vi "VI Tree.vi"   [LabVIEW 2016, in "Tektronix DPO MSO 2000 4000 Series.lvlib"]
doc: "This is the instrument driver for Tektronix DPO (2k, 3k, 4k), MSO (2k, 3k, 4k), and MDO. The VI Tree displays all the user-callable VIs of the instrument driver in an organized table."
uses:
  Tektronix DPO MSO 2000 4000 Series.lvlib
  Configure/Configure Probe (Auxiliary).vi
  Data/Data_Low Level/Fetch Waveform (Waveform Data Type).vi
  Configure/Configure Math (Dual).vi
  Configure/Configure Trigger (USB).vi
  Configure/Configure Bus Source (I2C).vi
  Data/Read (Multiple Waveforms).vi
panel:
  # "(C) 2006 - 2016. National Instruments Corporation. ALL RIGHTS RESERVED."
  # "SEE DIAGRAM\nFOR VI TREE."
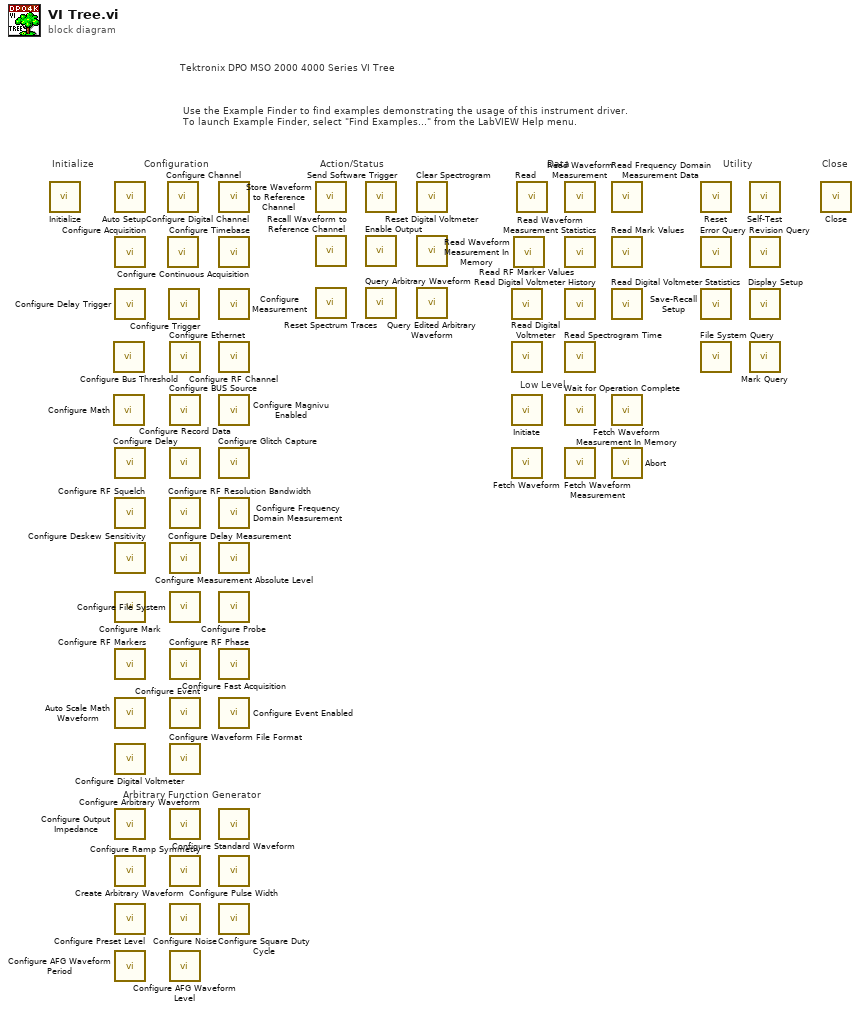
[diagram p0: block diagram]
diagram:
  # "Arbitrary Function Generator"
  # "Tektronix DPO MSO 2000 4000 Series VI Tree"
  # "Use the Example Finder to find examples demonstrating the usage of this instrument driver.\nTo launch Example Finder, select \"Find Examples...\" from the LabVIEW Help menu."
  # "Low Level"
  # "Action/Status"
  # "Configuration"
  # "Utility"
  # "Data"
  # "Close"
  # "Initialize"
  n1 = call "Initialize.vi"() -> ()  [unwired: 10 in, 2 out]
  n2 = call "Configure Bus Threshold.vi"() -> ()  [unwired: 10 in, 2 out]
  n3 = call-poly "Configure Math.vi"() -> ()  [unwired: 10 in, 2 out]
  n4 = call "Auto Setup.vi"() -> ()  [unwired: 10 in, 2 out]
  n5 = call "Configure Acquisition.vi"() -> ()  [unwired: 10 in, 2 out]
  n6 = call "Configure Delay Trigger.vi"() -> ()  [unwired: 14 in, 2 out]
  n7 = call "Configure Delay.vi"() -> ()  [unwired: 10 in, 2 out]
  n8 = call "Configure RF Squelch.vi"() -> ()  [unwired: 10 in, 2 out]
  n9 = call "Configure Deskew Sensitivity.vi"() -> ()  [unwired: 10 in, 2 out]
  n10 = call "Configure Mark.vi"() -> ()  [unwired: 10 in, 2 out]
  n11 = call "Configure RF Markers.vi"() -> ()  [unwired: 14 in, 2 out]
  n12 = call "Auto Scale Math Waveform.vi"() -> ()  [unwired: 10 in, 2 out]
  n13 = call "Configure Digital Voltmeter.vi"() -> ()  [unwired: 10 in, 2 out]
  n14 = call "Configure Output Impedance.vi"() -> ()  [unwired: 10 in, 2 out]
  n15 = call "Create Arbitrary Waveform.vi"() -> ()  [unwired: 10 in, 2 out]
  n16 = call "Configure Preset Level.vi"() -> ()  [unwired: 10 in, 2 out]
  n17 = call "Configure AFG Waveform Period.vi"() -> ()  [unwired: 10 in, 2 out]
  n18 = call "Configure Channel.vi"() -> ()  [unwired: 14 in, 2 out]
  n19 = call "Configure Continuous Acquisition.vi"() -> ()  [unwired: 10 in, 2 out]
  n20 = call-poly "Configure Trigger.vi"() -> ()  [unwired: 14 in, 2 out]
  n21 = call "Configure Ethernet.vi"() -> ()  [unwired: 14 in, 2 out]
  n22 = call-poly "Configure BUS Source.vi"() -> ()  [unwired: 14 in, 2 out]
  n23 = call "Configure Record Data.vi"() -> ()  [unwired: 10 in, 2 out]
  n24 = call "Configure RF Resolution Bandwidth.vi"() -> ()  [unwired: 14 in, 2 out]
  n25 = call "Configure Delay Measurement.vi"() -> ()  [unwired: 10 in, 2 out]
  n26 = call "Configure File System.vi"() -> ()  [unwired: 10 in, 2 out]
  n27 = call "Configure RF Phase.vi"() -> ()  [unwired: 10 in, 2 out]
  n28 = call "Configure Event.vi"() -> ()  [unwired: 10 in, 2 out]
  n29 = call "Configure Waveform File Format.vi"() -> ()  [unwired: 10 in, 2 out]
  n30 = call "Configure Arbitrary Waveform.vi"() -> ()  [unwired: 10 in, 2 out]
  n31 = call "Configure Ramp Symmetry.vi"() -> ()  [unwired: 10 in, 2 out]
  n32 = call "Configure Noise.vi"() -> ()  [unwired: 10 in, 2 out]
  n33 = call "Configure AFG Waveform Level.vi"() -> ()  [unwired: 10 in, 2 out]
  n34 = call "Configure Digital Channel.vi"() -> ()  [unwired: 10 in, 2 out]
  n35 = call "Configure Timebase.vi"() -> ()  [unwired: 10 in, 2 out]
  n36 = call "Configure Measurement.vi"() -> ()  [unwired: 14 in, 2 out]
  n37 = call "Configure RF Channel.vi"() -> ()  [unwired: 18 in, 2 out]
  n38 = call "Configure Magnivu Enabled.vi"() -> ()  [unwired: 10 in, 2 out]
  n39 = call "Configure Glitch Capture.vi"() -> ()  [unwired: 14 in, 2 out]
  n40 = call "Configure Frequency Domain Measurement.vi"() -> ()  [unwired: 14 in, 2 out]
  n41 = call "Configure Measurement Absolute Level.vi"() -> ()  [unwired: 14 in, 2 out]
  n42 = call-poly "Configure Probe.vi"() -> ()  [unwired: 10 in, 2 out]
  n43 = call "Configure Fast Acquisition.vi"() -> ()  [unwired: 10 in, 2 out]
  n44 = call "Configure Event Enabled.vi"() -> ()  [unwired: 10 in, 2 out]
  n45 = call "Configure Standard Waveform.vi"() -> ()  [unwired: 10 in, 2 out]
  n46 = call "Configure Pulse Width.vi"() -> ()  [unwired: 10 in, 2 out]
  n47 = call "Configure Square Duty Cycle.vi"() -> ()  [unwired: 10 in, 2 out]
  n48 = call "Store Waveform to Reference Channel.vi"() -> ()  [unwired: 10 in, 2 out]
  n49 = call "Recall Waveform to Reference Channel.vi"() -> ()  [unwired: 10 in, 2 out]
  n50 = call "Reset Spectrum Traces.vi"() -> ()  [unwired: 10 in, 2 out]
  n51 = call "Send Software Trigger.vi"() -> ()  [unwired: 10 in, 2 out]
  n52 = call "Enable Output.vi"() -> ()  [unwired: 10 in, 2 out]
  n53 = call "Query Arbitrary Waveform.vi"() -> ()  [unwired: 8 in, 4 out]
  n54 = call "Clear Spectrogram.vi"() -> ()  [unwired: 10 in, 2 out]
  n55 = call "Reset Digital Voltmeter.vi"() -> ()  [unwired: 10 in, 2 out]
  n56 = call "Query Edited Arbitrary Waveform.vi"() -> ()  [unwired: 8 in, 4 out]
  n57 = call "Read RF Marker Values.vi"() -> ()  [unwired: 11 in, 5 out]
  n58 = call "Read Digital Voltmeter.vi"() -> ()  [unwired: 8 in, 4 out]
  n59 = call "Initiate.vi"() -> ()  [unwired: 10 in, 2 out]
  n60 = call-poly "Fetch Waveform.vi"() -> ()  [unwired: 9 in, 3 out]
  n61 = call "Read Waveform Measurement In Memory.vi"() -> ()  [unwired: 9 in, 3 out]
  n62 = call-poly "Read.vi"() -> ()  [unwired: 9 in, 3 out]
  n63 = call "Read Waveform Measurement.vi"() -> ()  [unwired: 9 in, 3 out]
  n64 = call "Read Waveform Measurement Statistics.vi"() -> ()  [unwired: 6 in, 6 out]
  n65 = call "Read Digital Voltmeter History.vi"() -> ()  [unwired: 7 in, 5 out]
  n66 = call "Read Spectrogram Time.vi"() -> ()  [unwired: 8 in, 4 out]
  n67 = call "Wait for Operation Complete.vi"() -> ()  [unwired: 10 in, 2 out]
  n68 = call "Fetch Waveform Measurement.vi"() -> ()  [unwired: 9 in, 3 out]
  n69 = call "Read Frequency Domain Measurement Data.vi"() -> ()  [unwired: 7 in, 5 out]
  n70 = call "Read Mark Values.vi"() -> ()  [unwired: 9 in, 3 out]
  n71 = call "Read Digital Voltmeter Statistics.vi"() -> ()  [unwired: 8 in, 4 out]
  n72 = call "Fetch Waveform Measurement In Memory.vi"() -> ()  [unwired: 9 in, 3 out]
  n73 = call "Abort.vi"() -> ()  [unwired: 10 in, 2 out]
  n74 = call "Reset.vi"() -> ()  [unwired: 10 in, 2 out]
  n75 = call "Error Query.vi"() -> ()  [unwired: 8 in, 4 out]
  n76 = call "Save-Recall Setup.vi"() -> ()  [unwired: 10 in, 2 out]
  n77 = call "File System Query.vi"() -> ()  [unwired: 6 in, 6 out]
  n78 = call "Self-Test.vi"() -> ()  [unwired: 8 in, 4 out]
  n79 = call "Revision Query.vi"() -> ()  [unwired: 8 in, 4 out]
  n80 = call "Display Setup.vi"() -> ()  [unwired: 14 in, 2 out]
  n81 = call "Mark Query.vi"() -> ()  [unwired: 5 in, 7 out]
  n82 = call "Close.vi"() -> ()  [unwired: 11 in, 1 out]
